vi "Theil-Sen_2010.vi"(4 "Aligning array sizes? (T)":bool=TRUE, 6 "error in (no error)":errorcluster, 7 "Sen parameter? (F)":bool, 8 "input_Y":dbl[](array[numeric]), 9 "input_X":dbl[](array[numeric])) -> (0 "error out":errorcluster, 1 "b":dbl format="%.2e", 2 "m":dbl format="%.6g", 3 "output_Y":dbl[](array[numeric]))   [LabVIEW 2010]
doc: "The Theil–Sen estimator of a set of two-dimensional points (xi, yi) is the median m of the slopes (yj - yi)/(xj - xi) determined by all pairs of sample points. Sen extended this definition to handle the case in which two data points have the same x coordinate. In Sen's definition, one takes the median of the slopes defined only from pairs of points having distinct x coordinates.\nOnce the slope m has been determined, one may determine a line from the sample points by setting the y-intercept b to be the median of the values yi - mxi. The fit line is then the line y = mx + b with coefficients m and b in slope–intercept form."
uses:
  <vilib>/Analysis/NI_AALBase.lvlib
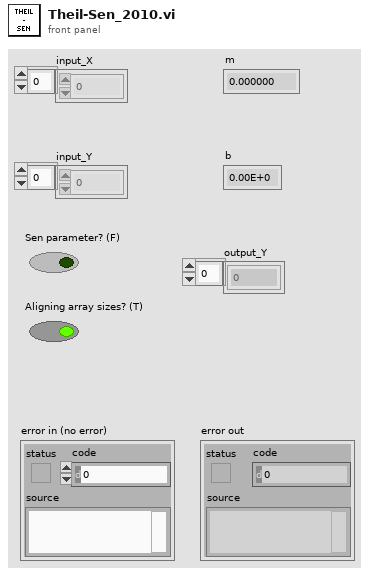
[diagram p1: front panel]
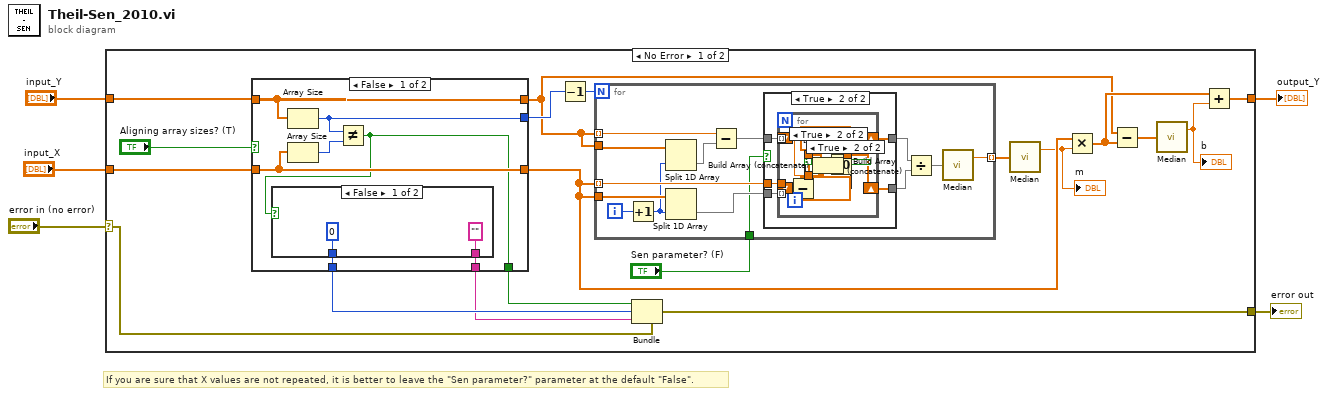
[diagram p0: block diagram]
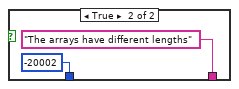
[diagram p2: hidden frame]
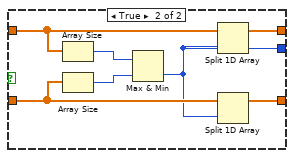
[diagram p3: hidden frame]
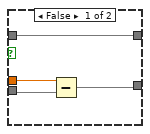
[diagram p4: hidden frame]
diagram:
  # "If you are sure that X values are not repeated, it is better to leave the \"Sen parameter?\" parameter at the default \"False\"."
  n1 = case shown="No Error" "error in (no error)" {
    selector: "error in (no error)" -> [w10 w86]
    tunnel: "input_X" -> [w24 _]
    tunnel: "input_Y" -> [w22 w85]
    tunnel: [w13 w86] -> w3
    tunnel: [w9 w85] -> w1
    frame No Error {
      n2 = case shown="False" "Aligning array sizes? (T)" {
        tunnel: w24 -> [w31 w40]
        tunnel: [w31 w39] -> w23
        tunnel: w22 -> [w30 w38]
        tunnel: [w30 w37] -> w6
        tunnel: [w26 _] -> w14
        tunnel: [w28 _] -> w12
        tunnel: [w27 _] -> w11
        tunnel: [w25 w36] -> w8
        frame False {
          n3 = Array Size(array=w30) -> (size(s)=w25:i32)
          n4 = Array Size(array=w31) -> (size(s)=w29:i32)
          n5 = Not Equal?(x=w25, y=w29) -> (x != y?=w26:bool)
          n6 = case shown="False" w26 {
            tunnel: [0 -20002] -> w28
            tunnel: ["" "The arrays have different lengths"] -> w27
            frame False {
            }
            frame True {
            }
          }
        }
        frame True {
          n7 = Array Size(array=w38) -> (size(s)=w42:i32)
          n8 = Array Size(array=w40) -> (size(s)=w41:i32)
          n9 = Max & Min(x=w42, y=w41) -> (min(x,y)=w36:i32)  [unwired: 1 out]
          n10 = Split 1D Array(array=w38, index=w36) -> (first subarray=w37:dbl[])  [unwired: 1 out]
          n11 = Split 1D Array(array=w40, index=w36) -> (first subarray=w39:dbl[])  [unwired: 1 out]
        }
      }
      n12 = Decrement(x=w8) -> (x-1=w21:i32)
      n13 = for {
        N: w21 -> [_]
        tunnel: w23 -> [w54] mode=indexing
        tunnel: w6 -> [w55]
        tunnel: w23 -> [w56]
        tunnel: [w48] -> w20 mode=indexing
        tunnel: "Sen parameter? (F)" -> [w44]
        tunnel: w6 -> [w43] mode=indexing
        i -> [w50]
        n14 = Increment(x=w50) -> (x+1=w49:i32)
        n15 = Split 1D Array(array=w55, index=w49) -> (second subarray=w52:dbl[])  [unwired: 1 out]
        n16 = Split 1D Array(array=w56, index=w49) -> (second subarray=w53:dbl[])  [unwired: 1 out]
        n17 = Subtract(x=w43, y=w52) -> (x-y=w46:dbl[])
        n18 = case shown="True" w44 {
          tunnel: w54 -> [w59 w67]
          tunnel: w53 -> [w58 w66]
          tunnel: [w57 w65] -> w47
          tunnel: w46 -> [w60 w64]
          tunnel: [w60 w63] -> w45
          frame False {
            n19 = Subtract(x=w59, y=w58) -> (x-y=w57:dbl[])
          }
          frame True {
            n20 = for {
              tunnel: w67 -> [w76]
              tunnel: w66 -> [w75] mode=indexing
              tunnel: w64 -> [w74] mode=indexing
              shift-right: [w70] -> w65
              shift-left: dbl[] [] ("Array") -> [w71]
              shift-right: [w68] -> w63
              shift-left: dbl[] [] ("Array") -> [w69]
              n21 = Subtract(x=w76, y=w75) -> (x-y=w72:dbl)
              n22 = Not Equal To 0?(x=w72) -> (x != 0?=w73:bool)
              n23 = case shown="True" w73 {
                tunnel: w69 -> [w77 w79]
                tunnel: w74 -> [_ w78]
                tunnel: [w77 w80] -> w68
                frame False {
                }
                frame True {
                  n24 = Build Array (concatenate)(w79, w78) -> (w80:dbl[])
                }
              }
              n25 = case shown="True" w73 {
                tunnel: w71 -> [w81 w83]
                tunnel: w72 -> [_ w82]
                tunnel: [w81 w84] -> w70
                frame False {
                }
                frame True {
                  n26 = Build Array (concatenate)(w83, w82) -> (w84:dbl[])
                }
              }
            }
          }
        }
        n27 = Divide(x=w45, y=w47) -> (x/y=w51:dbl[])
        n28 = call <vilib>:"Median.vi"("X"=w51) -> ("median"=w48:dbl)  [unwired: 1 out]
      }
      n29 = Bundle(cluster=w10, "status"=w14, "code"=w12, "source"=w11) -> (w13:errorcluster)
      n30 = call <vilib>:"Median.vi"("X"=w20) -> ("median"=w17:dbl)  [unwired: 1 out]
      "m" <- w17
      n31 = Multiply(x=w23, y=w17) -> (x*y=w18:dbl[])
      n32 = Subtract(x=w6, y=w18) -> (x-y=w19:dbl[])
      n33 = call <vilib>:"Median.vi"("X"=w19) -> ("median"=w16:dbl)  [unwired: 1 out]
      "b" <- w16
      n34 = Add(x=w18, y=w16) -> (x+y=w9:dbl[])
    }
    frame Error {
    }
  }
  "error out" <- w3
  "output_Y" <- w1
